vi "set_resolution.vi"(8 "error in (no error)":errorcluster, 9 "y resolution":i32, 10 "x resolution":i32, 11 "DL090211FrameImageAssembler.lvclass in":refnum<class "ImageAssemblerDL090211Frame.lvclass">) -> (0 "error out":errorcluster, 3 "DL090211FrameImageAssembler.lvclass out":refnum<class "ImageAssemblerDL090211Frame.lvclass">)   [LabVIEW 2010, in "ImageAssemblerDL090211Frame.lvclass"]
uses:
  ImageAssemblerDL090211Frame.lvclass
  ImageAssemblerDL090211Frame.lvclass/ImageAssemblerDL090211Frame.ctl
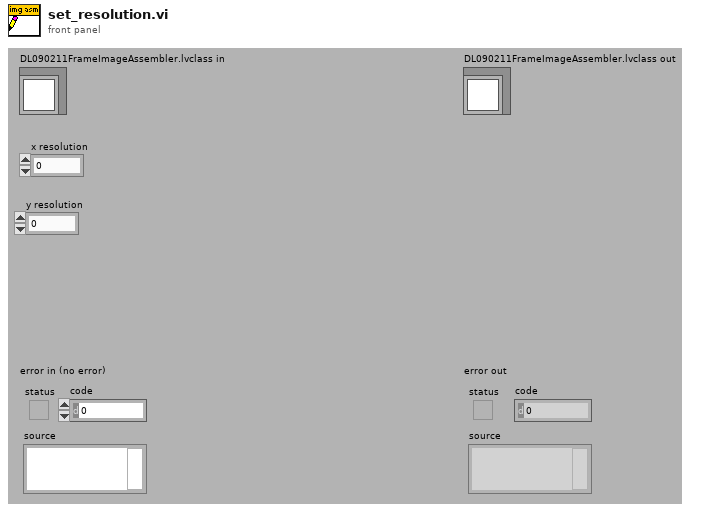
[diagram p1: front panel]
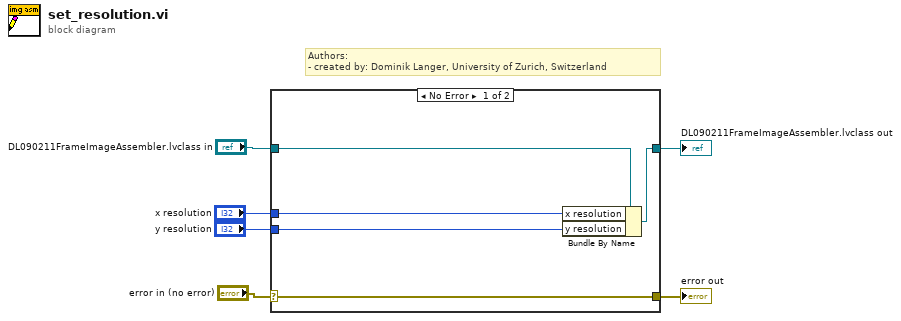
[diagram p0: block diagram]
diagram:
  # "Authors: \n- created by: Dominik Langer, University of Zurich, Switzerland"
  n1 = case shown="No Error" "error in (no error)" {
    selector: "error in (no error)" -> [w11 w12]
    tunnel: [w11 w12] -> w5
    tunnel: [w9 w13] -> w3
    tunnel: "DL090211FrameImageAssembler.lvclass in" -> [w10 w13]
    tunnel: "x resolution" -> [w8 _]
    tunnel: "y resolution" -> [w7 _]
    frame No Error {
      n2 = Bundle By Name(cluster=w10, "x resolution"=w8, "y resolution"=w7) -> (w9:refnum<class "ImageAssemblerDL090211Frame.lvclass">)
    }
    frame Error {
    }
  }
  "error out" <- w5
  "DL090211FrameImageAssembler.lvclass out" <- w3
